vi "Write_data_to_file_time_sender_dtgn.vi"(8 "error in (no error)":errorcluster, 9 "Datagram number":u32, 10 "Sender number":u8, 11 "Byte Stream File in":refnum<file>) -> (0 "error out":errorcluster, 3 "Byte Stream File out":refnum<file>)   [LabVIEW 2013]
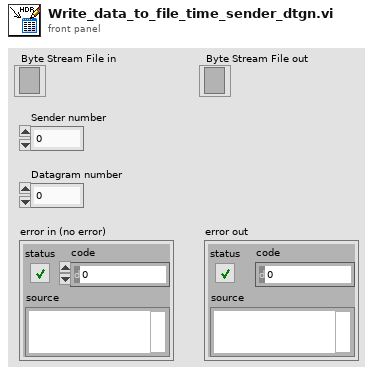
[diagram p1: front panel]
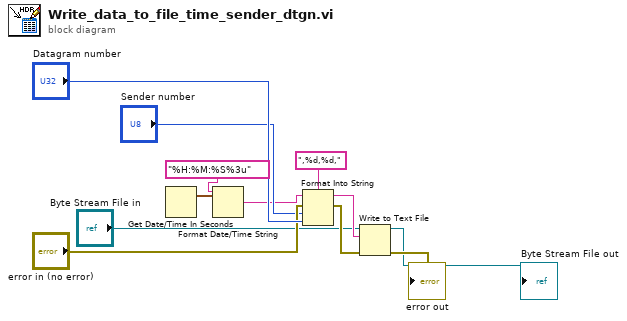
[diagram p0: block diagram]
diagram:
  n1 = Get Date/Time In Seconds() -> (seconds since 1Jan1904=w4:timestamp)
  n2 = Format Date/Time String(time format string (%c)="%H:%M:%S%3u", seconds (now)=w4) -> (date/time string=w7:string)  [unwired: 1 in]
  n3 = Format Into String(format string=",%d,%d,", initial string=w7, error in="error in (no error)", "Sender number", "Datagram number") -> (resulting string=w6:string, error out=w10:errorcluster)
  n4 = Write to Text File(file (use dialog)="Byte Stream File in", text=w6, error in=w10) -> (refnum out=→"Byte Stream File out":refnum<file>, error out=→"error out":errorcluster)  [unwired: 1 in, 1 out]
